vi "Top Level.vi"() -> ()   [LabVIEW 2015]
uses:
  Admin_Actor/Admin_Actor/Admin_Actor.lvclass
  Member_Actor/Member_Actor/Member_Actor.lvclass
  <vilib>/Utility/config.llb/Read Key (Boolean).vi
  Admin_Actor/Setting/g_setting.vi
  <vilib>/Utility/config.llb/Write Key (Boolean).vi
  Login/Public Methods/Login Main Panel.vi
  User_Actor/User_Actor/User_Actor.lvclass
  Login/Login.lvclass
  <vilib>/Utility/config.llb/NI_LVConfig.lvlib
panel:
  in  "error in (no error)":errorcluster
  in  "Member":bool
  in  "Admin":bool
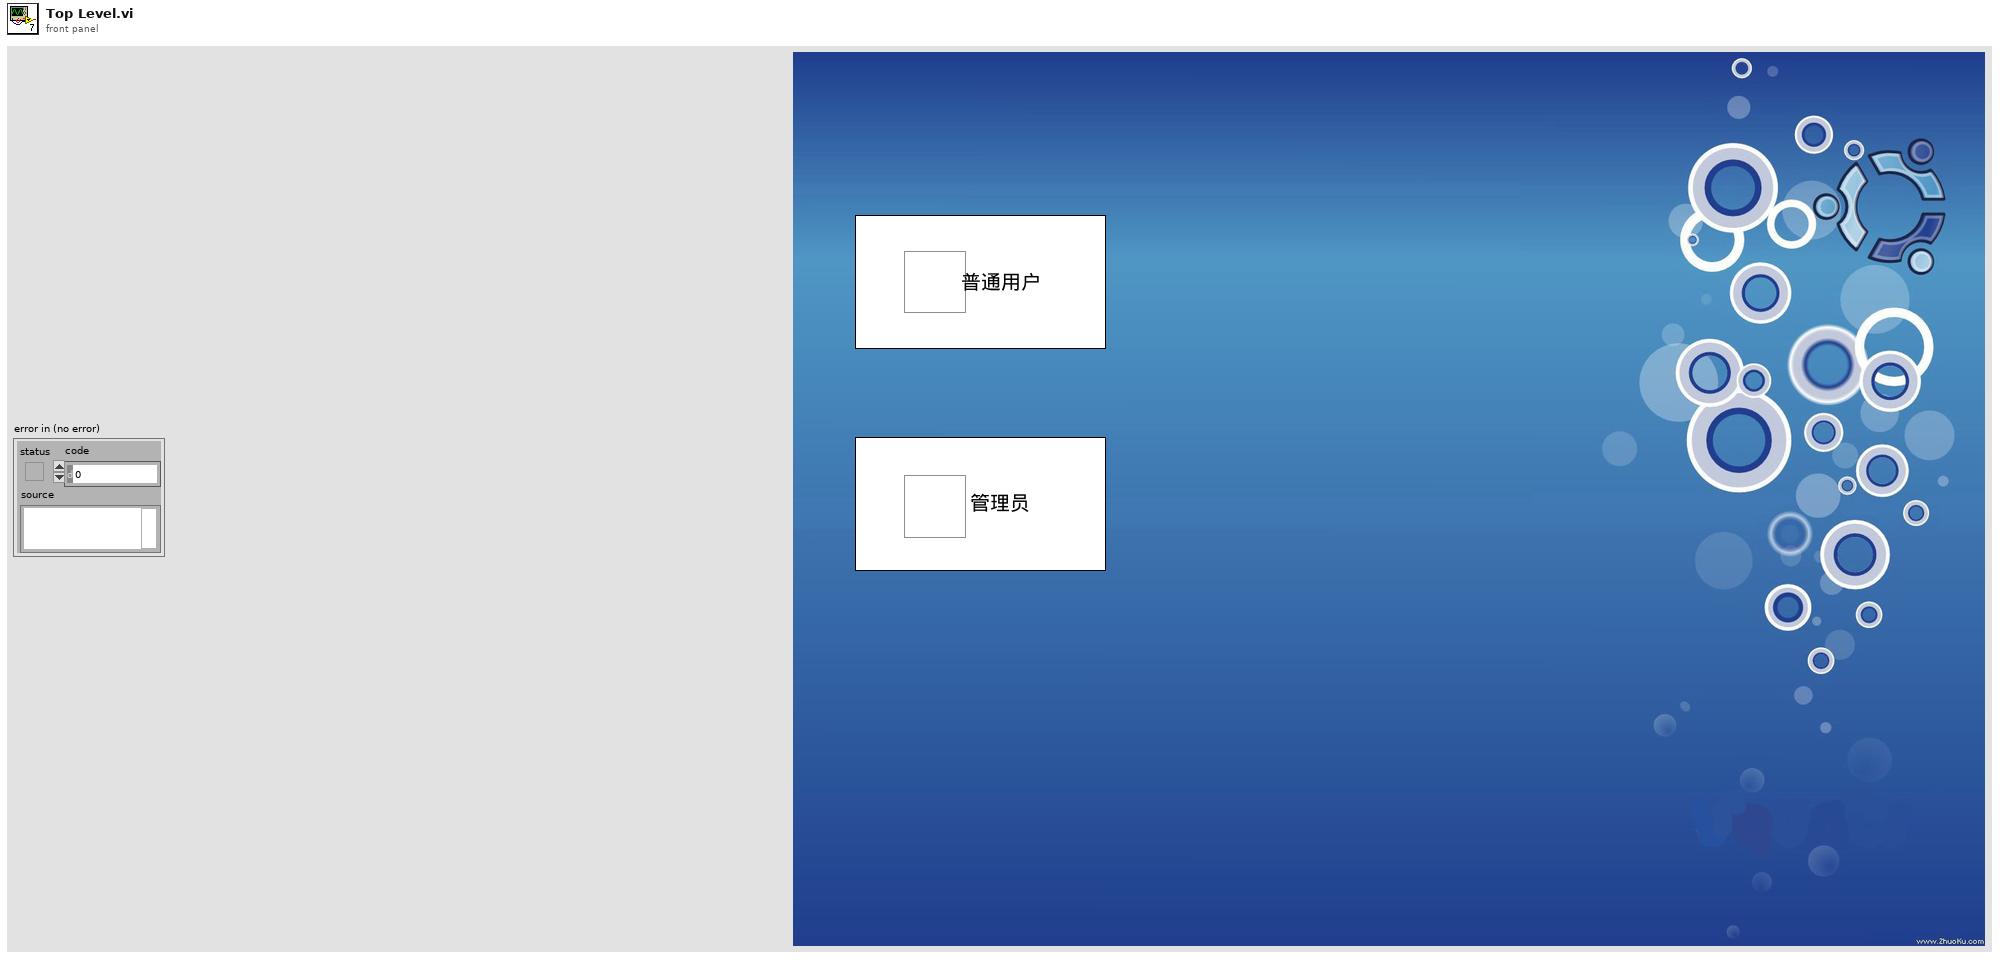
[diagram p1: front panel]
types:
  T1 = typedef "NI_LVConfig.lvlib/Config Data RefNum.ctl" = refnum<k1>
  T2 = enum32{"Invalid", "Standard", "Closed", "Hidden", "Minimized", "Maximized"}
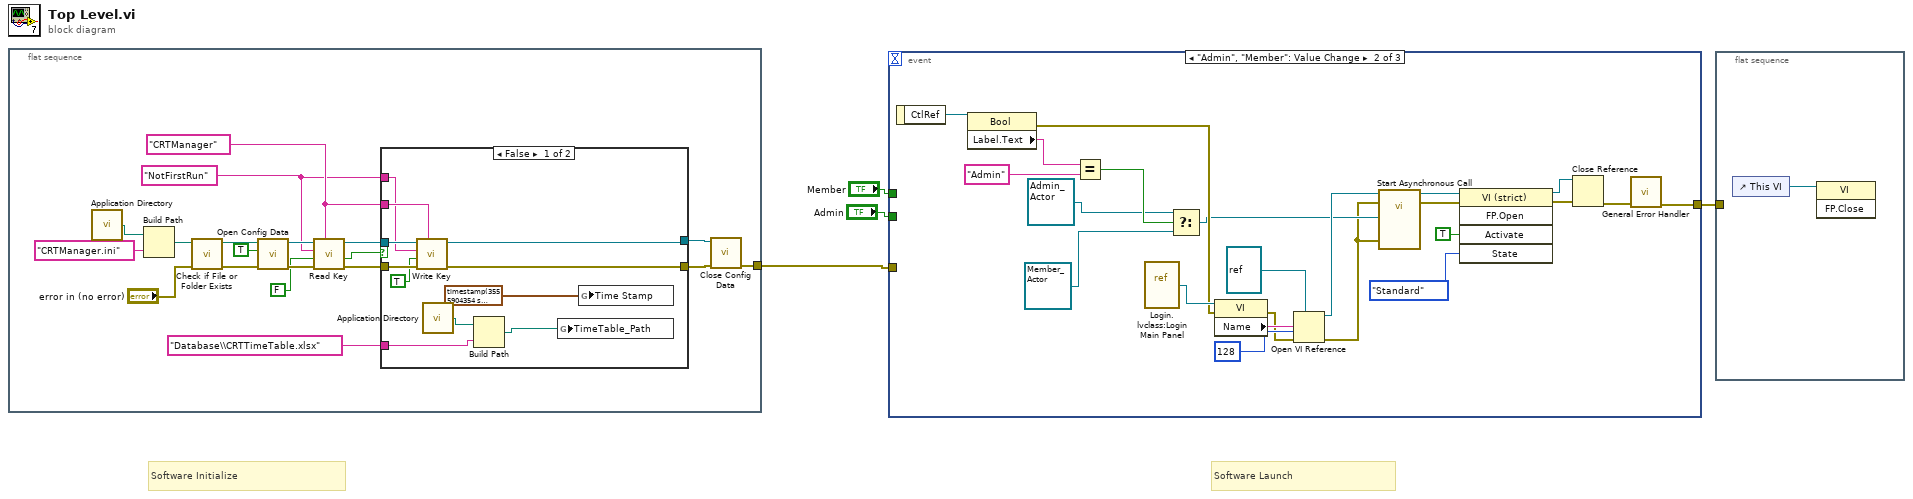
[diagram p0: block diagram]
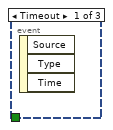
[diagram p3: hidden frame]
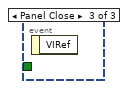
[diagram p4: hidden frame]
diagram:
  # "Software Launch"
  # "Software Initialize"
  n1 = flat-sequence {
    tunnel: [w5] -> w1
    frame #0 {
      w9 = "NotFirstRun" ("key")
      w10 = "CRTManager" ("section")
      n2 = call <vilib>:"Application Directory.vi"() -> ("Application Directory"=w23:path)
      n3 = Build Path(base path=w23, name or relative path="CRTManager.ini") -> (appended path=w21:path)
      n4 = call <vilib>:"Check if File or Folder Exists.vi"("error in (no error)"="error in (no error)", "path"=w21) -> ("error out"=w18:errorcluster, "dup path"=w19:path)  [unwired: 7 in, 1 out]
      n5 = call <vilib>:"Open Config Data.vi"("error in (no error)"=w18, "create file if necessary (T)"=TRUE, "configuration file path"=w19) -> ("error out"=w15:errorcluster, "refnum"=w16:T1)  [unwired: 6 in, 1 out]
      n6 = call-poly <vilib>:"Read Key.vi"("section"=w10, "error in (no error)"=w15, "default value"=FALSE, "key"=w9, "refnum"=w16) -> ("error out"=w13:errorcluster, "value"=w11:bool, "refnum out"=w14:T1)  [unwired: 3 in, 1 out]
      n7 = case shown="False" w11 {
        tunnel: w14 -> [w30 w36]
        tunnel: w13 -> [w29 w35]
        tunnel: w10 -> [w28 _]
        tunnel: w9 -> [w27 _]
        tunnel: [w24 w36] -> w8
        tunnel: [w25 w35] -> w7
        tunnel: "Database\\CRTTimeTable.xlsx" -> [w32 _]
        frame False {
          n8 = call-poly <vilib>:"Write Key.vi"("section"=w28, "error in (no error)"=w29, "value"=TRUE, "key"=w27, "refnum"=w30) -> ("error out"=w25:errorcluster, "refnum out"=w24:T1)  [unwired: 4 in, 1 out]
          n9 = call <vilib>:"Application Directory.vi"() -> ("Application Directory"=w33:path)
          n10 = Build Path(base path=w33, name or relative path=w32) -> (appended path=w31:path)
          n11 = global write "g_setting.vi" "TimeTable_Path"(w31) -> ()
          n12 = global write "g_setting.vi" "Time Stamp"(timestamp(3555904354.214689 s since 1904-01-01) ("Time Stamp")) -> ()
        }
        frame True {
        }
      }
      n13 = call <vilib>:"Close Config Data.vi"("error in (no error)"=w7, "refnum"=w8) -> ("error out"=w5:errorcluster)  [unwired: 8 in, 1 out]
    }
  }
  n14 = event shown="[1] \"Admin\", \"Member\": Value Change" {
    selector: _ -> [_ _ _]
    dyn-events: _ -> [_ _ _]
    timeout: _ -> [_ _ _]
    tunnel: "Member" -> [_ _ _]
    tunnel: "Admin" -> [_ _ _]
    tunnel: [_ w43 _] -> w2
    tunnel: w1 -> [_ _ _]
    event Timeout {
      n15 = event-data() -> ()  [unwired: 1 in, 3 out]
    }
    event "Admin", "Member": Value Change {
      n16 = event-data() -> ("CtlRef"=w59:refnum<vi>)  [unwired: 1 in]
      n17 = property class="Bool"(reference=w59) -> (error out=w49:errorcluster, "Label.Text"=w58:string)  [unwired: 1 in, 1 out]
      n18 = Equal?(x=w58, y="Admin") -> (x = y?=w56:bool)
      n19 = vi-ref "Login.lvclass:Login Main Panel.vi"() -> (w53:refnum<vi>)
      n20 = Select(t=refnum<class "Admin_Actor.lvclass"> refnum ("Admin_Actor.lvlib:Admin_Actor.lvclass"), s=w56, f=refnum<class "Member_Actor.lvclass"> refnum ("Member_Actor.lvlib:Member_Actor.lvclass")) -> (s? t:f=w46:refnum<class "User_Actor.lvclass">)
      n21 = property class="VI"(reference=w53, error in=w49) -> (error out=w48:errorcluster, "Name"=w52:string)  [unwired: 1 out]
      n22 = Open VI Reference(type specifier VI Refnum (for type only)=refnum<vi> refnum, vi path=w52, options=128, error in (no error)=w48) -> (vi reference=w47:refnum<vi>, error out=w45:errorcluster)  [unwired: 2 in]
      n23 = call-by-ref "Start Asynchronous Call"(reference=w47, error in=w45, 8:"error in (no error)"=w45, "User_Actor.lvclass"=w46) -> (reference out=w42:refnum<vi>, error out=w40:errorcluster)  [unwired: 9 in, 1 out]
      n24 = invoke class="VI (strict)" method="FP.Open"(reference=w42, error in=w40, "Activate"=TRUE ("Activate?"), "State"=T2."Standard") -> (reference out=w41:refnum<vi>, error out=w39:errorcluster)  [unwired: 1 in, 3 out]
      n25 = Close Reference(reference=w41, error in (no error)=w39) -> (error out=w44:errorcluster)
      n26 = call <vilib>:"General Error Handler.vi"("error in (no error)"=w44) -> ("error out"=w43:errorcluster)  [unwired: 10 in, 4 out]
    }
    event Panel Close {
      n27 = event-data() -> ()  [unwired: 1 in, 1 out]
    }
  }
  n28 = flat-sequence {
    tunnel: w2 -> [_]
    frame #0 {
      n29 = control-ref of="This VI"() -> (w60:refnum<vi>)
      n30 = invoke class="VI" method="FP.Close"(reference=w60) -> ()  [unwired: 2 in, 3 out]
    }
  }
